vi "Get SMS Attributes.vi"(8 "error in (no error)":errorcluster, 11 "SMS in":refnum<class "SMS.lvclass">) -> (0 "error out":errorcluster, 2 "SMS Attributes":T1[](array[typedef]), 3 "SMS out":refnum<class "SMS.lvclass">)   [LabVIEW 2015, in "NI_AWS_SNS.lvlib" / "SMS.lvclass"]
uses:
  SMS.lvclass
  SMS Attribute Value Pair.ctl
  SMS Attribute.ctl
  Core/HTTP Request/Request Options.ctl
  Core/HTTP Request/Name Value Pair.ctl
  Core/HTTP Request/Region handling.ctl
  Core/HTTP Request/URL formatting.ctl
  Core/HTTP Request/HTTP Request.lvclass
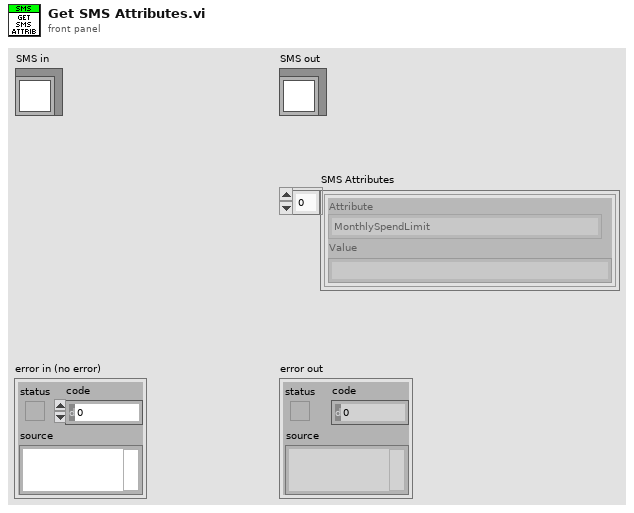
[diagram p1: front panel]
types:
  T1 = typedef "NI_AWS_SNS.lvlib/SMS.lvclass/SMS Attribute Value Pair.ctl" = cluster{"Attribute":T2, "Value":string}
  T2 = typedef "NI_AWS_SNS.lvlib/SMS.lvclass/SMS Attribute.ctl" = enum16{"MonthlySpendLimit", "DeliveryStatusIAMRole", "DeliveryStatusSuccessSamplingRate", "DefaultSenderID", "DefaultSMSType", "UsageReportS3Bucket"}
  T3 = typedef "NI_AWS_Core.lvlib/HTTP Request.lvclass/Name Value Pair.ctl" = cluster{"name":string, "value":string}
  T4 = typedef "NI_AWS_Core.lvlib/HTTP Request.lvclass/Request Options.ctl" = cluster{"request headers":T3[], "request parameters":T3[], "request body":string, "region handling":T5, "URL formatting":T6}
  T5 = typedef "NI_AWS_Core.lvlib/HTTP Request.lvclass/Region handling.ctl" = enum16{"use region everywhere", "use region (authentication only)", "use region (URL only)", "ignore region everwhere"}
  T6 = typedef "NI_AWS_Core.lvlib/HTTP Request.lvclass/URL formatting.ctl" = enum16{"region-", "region."}
  T7 = typedef "NI_AWS_Core.lvlib/HTTP Request.lvclass/Response.ctl" = cluster{"Headers":string, "Body":string}
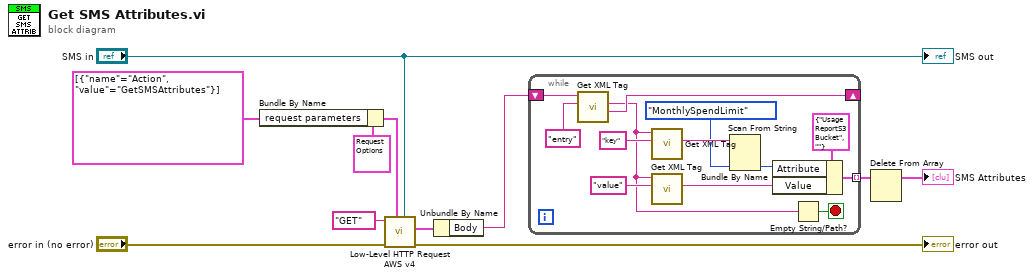
[diagram p0: block diagram]
diagram:
  n1 = Bundle By Name(cluster=T4 {"request headers"=[], "request parameters"=[], "request body"="", "region handling"=enum."use region everywhere", "URL formatting"=enum."region."} ("Request Options"), "request parameters"=T3[] [{"name"="Action", "value"="GetSMSAttributes"}]) -> (w6:T4)
  n2 = call "Low-Level HTTP Request AWS v4.vi"("AWS Core"="SMS in", "Request Options"=w6, "error in (no error)"="error in (no error)", "HTTP-Verb"="GET") -> ("error out"=→"error out":errorcluster, "Response"=w4:T7)  [unwired: 5 in, 1 out]
  n3 = Unbundle By Name(w4) -> ("Body"=w3:string)
  n4 = while {
    shift-right: [w23] -> _
    shift-left: w3 -> [w24]
    tunnel: [w18] -> w2 mode=indexing
    stop <- w16 stop-if-true
    n5 = call "Get XML Tag.vi"("Tag name"="entry", "XML String in"=w24) -> ("Remaining string"=w23:string, "Tag value"=w17:string)  [unwired: 5 in, 3 out]
    n6 = call "Get XML Tag.vi"("Tag name"="key", "XML String in"=w17) -> ("Tag value"=w14:string)  [unwired: 5 in, 4 out]
    n7 = call "Get XML Tag.vi"("Tag name"="value", "XML String in"=w17) -> ("Tag value"=w19:string)  [unwired: 5 in, 4 out]
    n8 = Scan From String(input string=w14, default 1=SMS_Attribute."MonthlySpendLimit" ("Attribute")) -> (output 1=w12:T2)  [unwired: 3 in, 3 out]
    n9 = Bundle By Name(cluster=T1 {"Attribute"=enum."UsageReportS3Bucket", "Value"=""} ("SMS Attribute Value Pair"), "Attribute"=w12, "Value"=w19) -> (w18:T1)
    n10 = Empty String/Path?(string/path=w17) -> (empty?=w16:bool)
  }
  n11 = Delete From Array(array=w2) -> (array with subset deleted=→"SMS Attributes":T1[])  [unwired: 2 in, 1 out]
  "SMS out" <- "SMS in"
